vi "read_access_codes_from_file.vi"(8 "error in (no error)":errorcluster, 11 "Paths":T1) -> (0 "error out":errorcluster, 3 "Codes":T2)   [LabVIEW 2016]
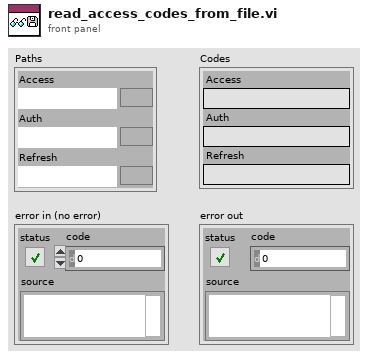
[diagram p1: front panel]
types:
  T1 = cluster{"Access":path, "Auth":path, "Refresh":path}
  T2 = cluster{"Access":string, "Auth":string, "Refresh":string}
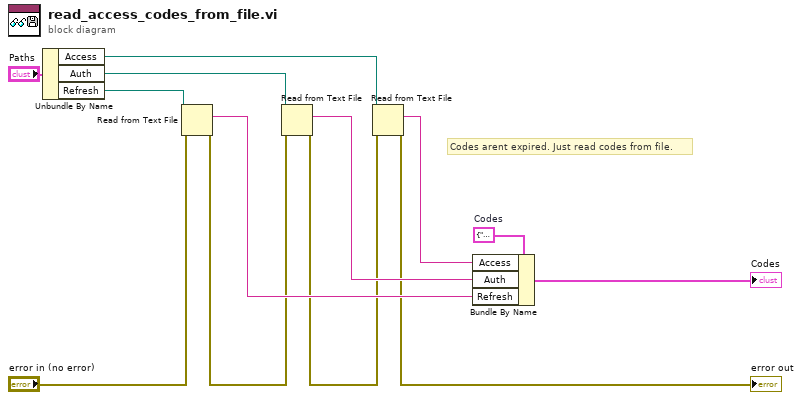
[diagram p0: block diagram]
diagram:
  w13 = T2 {"Access"="", "Auth"="", "Refresh"=""}  # Codes
  # "Codes arent expired. Just read codes from file."
  n1 = Unbundle By Name("Paths") -> ("Access"=w2:path, "Auth"=w3:path, "Refresh"=w4:path)
  n2 = Read from Text File(file (use dialog)=w4, error in="error in (no error)") -> (text=w10:string, error out=w6:errorcluster)  [unwired: 2 in, 2 out]
  n3 = Read from Text File(file (use dialog)=w3, error in=w6) -> (text=w11:string, error out=w7:errorcluster)  [unwired: 2 in, 2 out]
  n4 = Read from Text File(file (use dialog)=w2, error in=w7) -> (text=w9:string, error out=→"error out":errorcluster)  [unwired: 2 in, 2 out]
  n5 = Bundle By Name(cluster=w13, "Access"=w9, "Auth"=w11, "Refresh"=w10) -> (→"Codes":T2)
